vi "LCSS classification (edit).vi"(9 "cluster centers":string[](array[string])=["1 0 -1 1 -1 0 -4 1 -4 0 1", "2 0 -1 2 -1 0 -2 2 -2 0 2", "3 0 -3 3 -3 0 -2 3 -2 0 3", "4 0 -3 4 -3 0 -4 4 -4 0 4", "-1 1 -4 0 -4 4 -3 4 -4 0 -4 1 -1", "-1 2 -2 0 -2 3 -3 3 -2 0 -2 2 -1", "-4 1 -1 0 -1 2 -2 2 -1 0 -1 1 -4", "-4 4 -3 0 -3 3 -2 3 -3 0 -3 4 -4", "0 -4 1 -1 0 -3 3 -2 3 -3 0 -1 1 -4 0", "0 -4 4 -3 0 -1 2 -2 2 -1 0 -3 4 -4 0"], 11 "Patterns in":string[](array[string])=["0 4 0", "4 0 4", "0 4 0", "4 0 4", "0 4 0", "4 0 4", "0 4 0", "4 0 -2", "0 -2 3", "-2 3 0", "3 0 3", "0 3 0", "3 0 4", "0 4 0", "-2 0 1", "0 1 0", "1 0 -4", "0 -4 4", "-2 2 0", "2 0 -1", "0 -1 -4", "-1 -4 1", "-4 1 0", "1 0 3", "0 3 0", "-1 0 -1", "0 -1 2", "0 -1 1", "-1 1 0", "1 0 4", "0 4 0", "4 0 3", "0 3 -2", "3 -2 0", "-2 0 -2", "0 -2 3", "-2 3 -2", "3 -2 0", "-2 0 4", "0 4 0", "4 0 -2", "0 -2 2", "2 -1 0", "-1 0 4", "0 4 0", "4 0 2", "0 2 0", "2 0 -2", "0 -2 0", "1 -1 0", "-1 0 3", "0 3 0", "3 0 -4", "0 -4 4", "-4 4 -4", "4 -4 0", "2 -1 0", "-1 0 3", "0 3 -2", "3 -2 0", "-2 0 -3", "0 -3 0", "-3 0 3", "0 3 0", "3 0 -3", "0 -3 0", "0 4 0", "4 0 4", "0 4 -4", "4 -4 1", "-4 1 -1", "1 -1 0", "-1 0 -3", "0 -3 0", "-3 0 1", "0 1 -4", "1 -4 1", "-4 1 0", "1 0 4", "0 4 0", "4 0 -4", "0 -4 0", "-4 0 -4", "0 -4 4", "-4 4 -4", "4 -4 1", "0 -4 1", "-4 1 0", "1 0 -4", "0 -4 4", "0 4 0", "4 0 -2", "0 -2 2", "-2 2 -2", "2 -2 2", "-2 2 -2", "2 -2 2", "-2 2 -1", "2 -1 0", "-1 0 4", "0 4 0", "4 0 2", "0 2 0", "2 0 4", "0 4 0", "4 0 2", "0 2 -2", "2 -2 0", "-2 0 4", "1 0 -1", "0 -1 0", "-1 0 -1", "0 -1 0", "-1 0 1", "0 1 -1", "-2 2 -2", "2 -2 3", "1 0 -1", "0 -1 0", "-1 0 -1", "0 -1 2", "-1 2 0", "2 0 2", "0 2 -2", "2 -2 0", "-2 0 -4", "0 -4 0", "-2 2 0", "2 0 3", "0 3 -2", "3 -2 2", "1 -1 0", "-1 0 3", "0 4 0", "-2 0 1", "0 1 -4", "1 -4 0", "-4 0 -3", "0 -3 0", "1 0 -1", "0 -1 2", "-1 2 -1", "2 -1 1", "-1 1 -4", "-2 0 -1", "0 -1 1", "0 3 0", "3 0 3", "0 3 0", "3 0 3", "0 3 -2", "-4 0 -4", "0 -4 4", "0 4 0", "4 0 -4", "0 -4 0", "-4 0 -4", "-2 2 0", "2 0 4", "0 4 -4", "4 -4 0", "-4 0 2", "0 2 -2"]) -> (0 "Assigned cluster (0) unassigned":string[](array[string]), 1 "patterns in, distance values":string[][](array[string]), 2 "Assigned cluster 2nd method":string[](array[string]), 3 "Cluster element count":i32[](array[numeric]), 4 "Assigned cluster 3rd method 2":string[](array[string]))   [LabVIEW 2014]
panel:
  out "x = y?":bool[](array[boolean])
  out "Assigned cluster (0) unassigned 2":string[](array[string])
  out "Array 4":dbl[][](array[numeric])
  out "Array 3":dbl[][](array[numeric])
  out "Array 2":dbl[][](array[numeric])
  out "Array":dbl[][](array[numeric])
  out "L cluster centers":i32[](array[numeric])
  out "L sample":i32[](array[numeric])
  out "appended array":string[][](array[string])
  out "Distance values (LCS)":dbl[][](array[numeric])
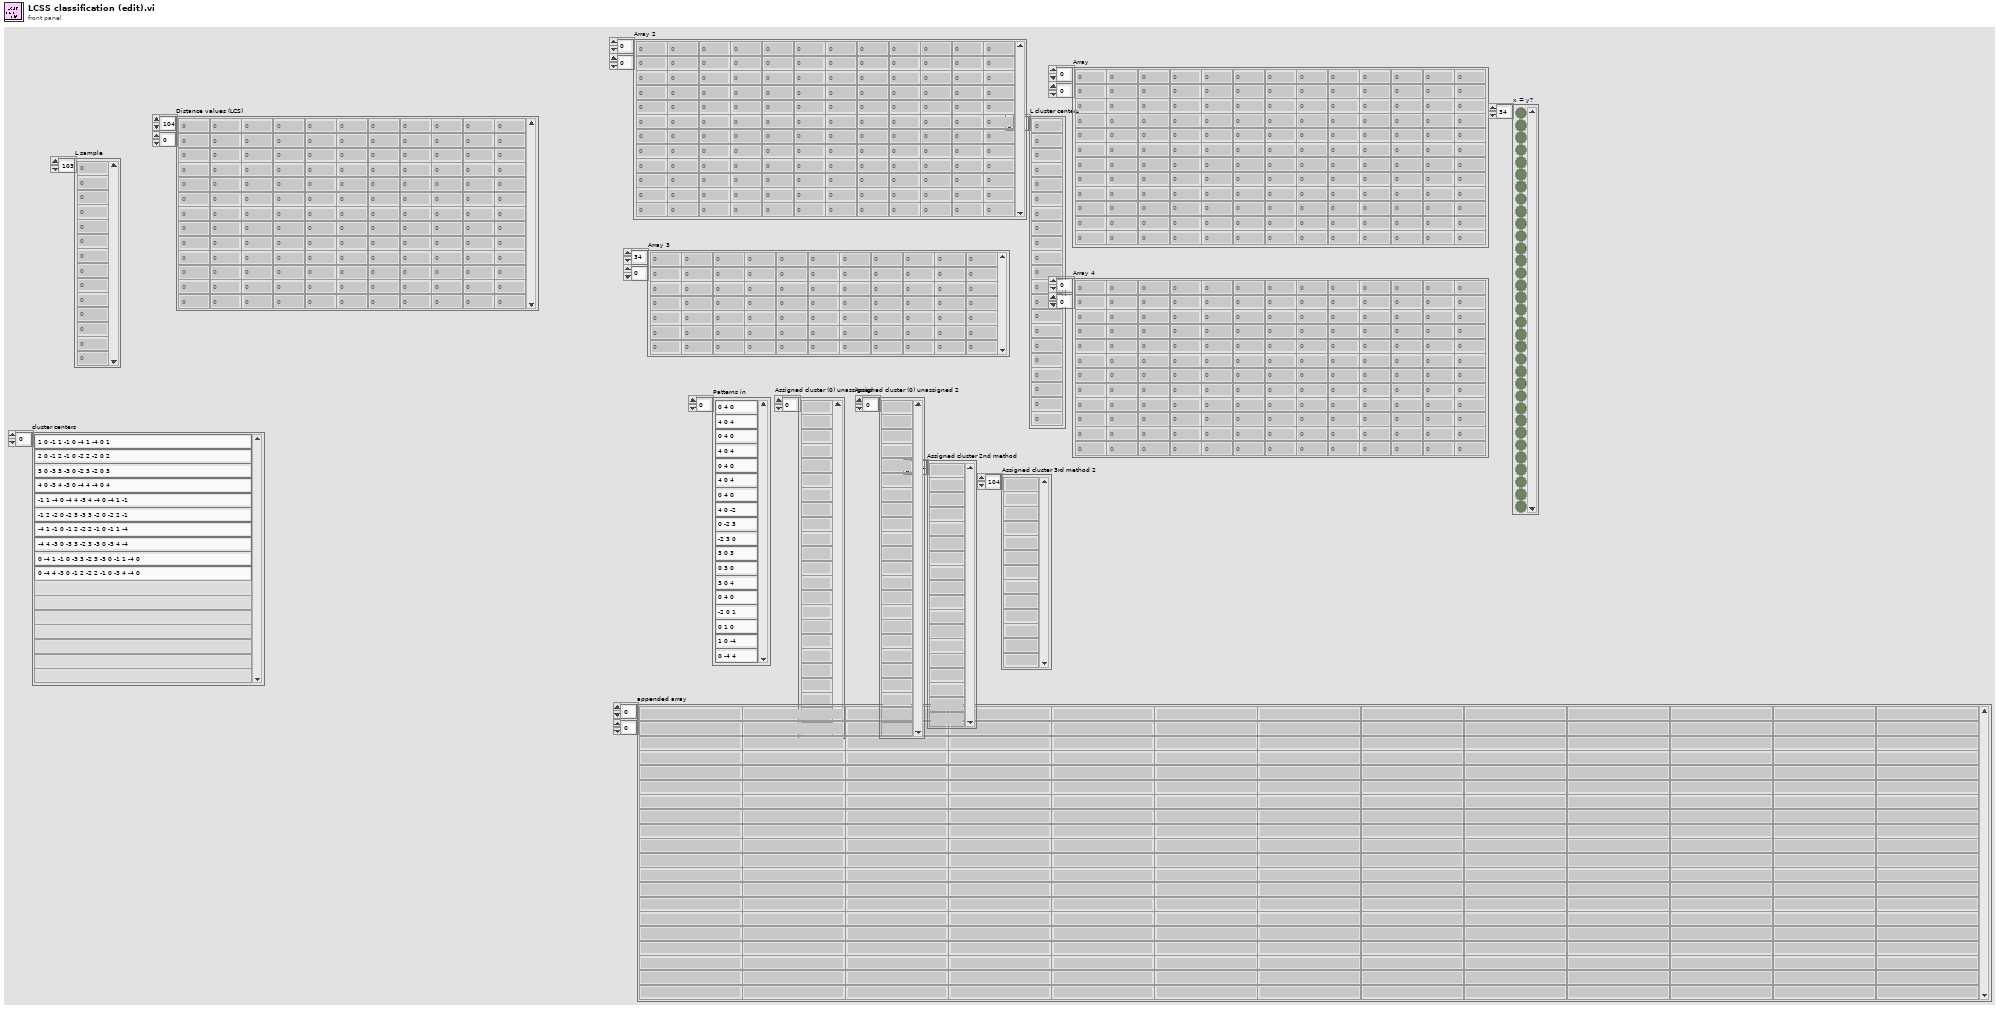
[diagram p1: front panel]
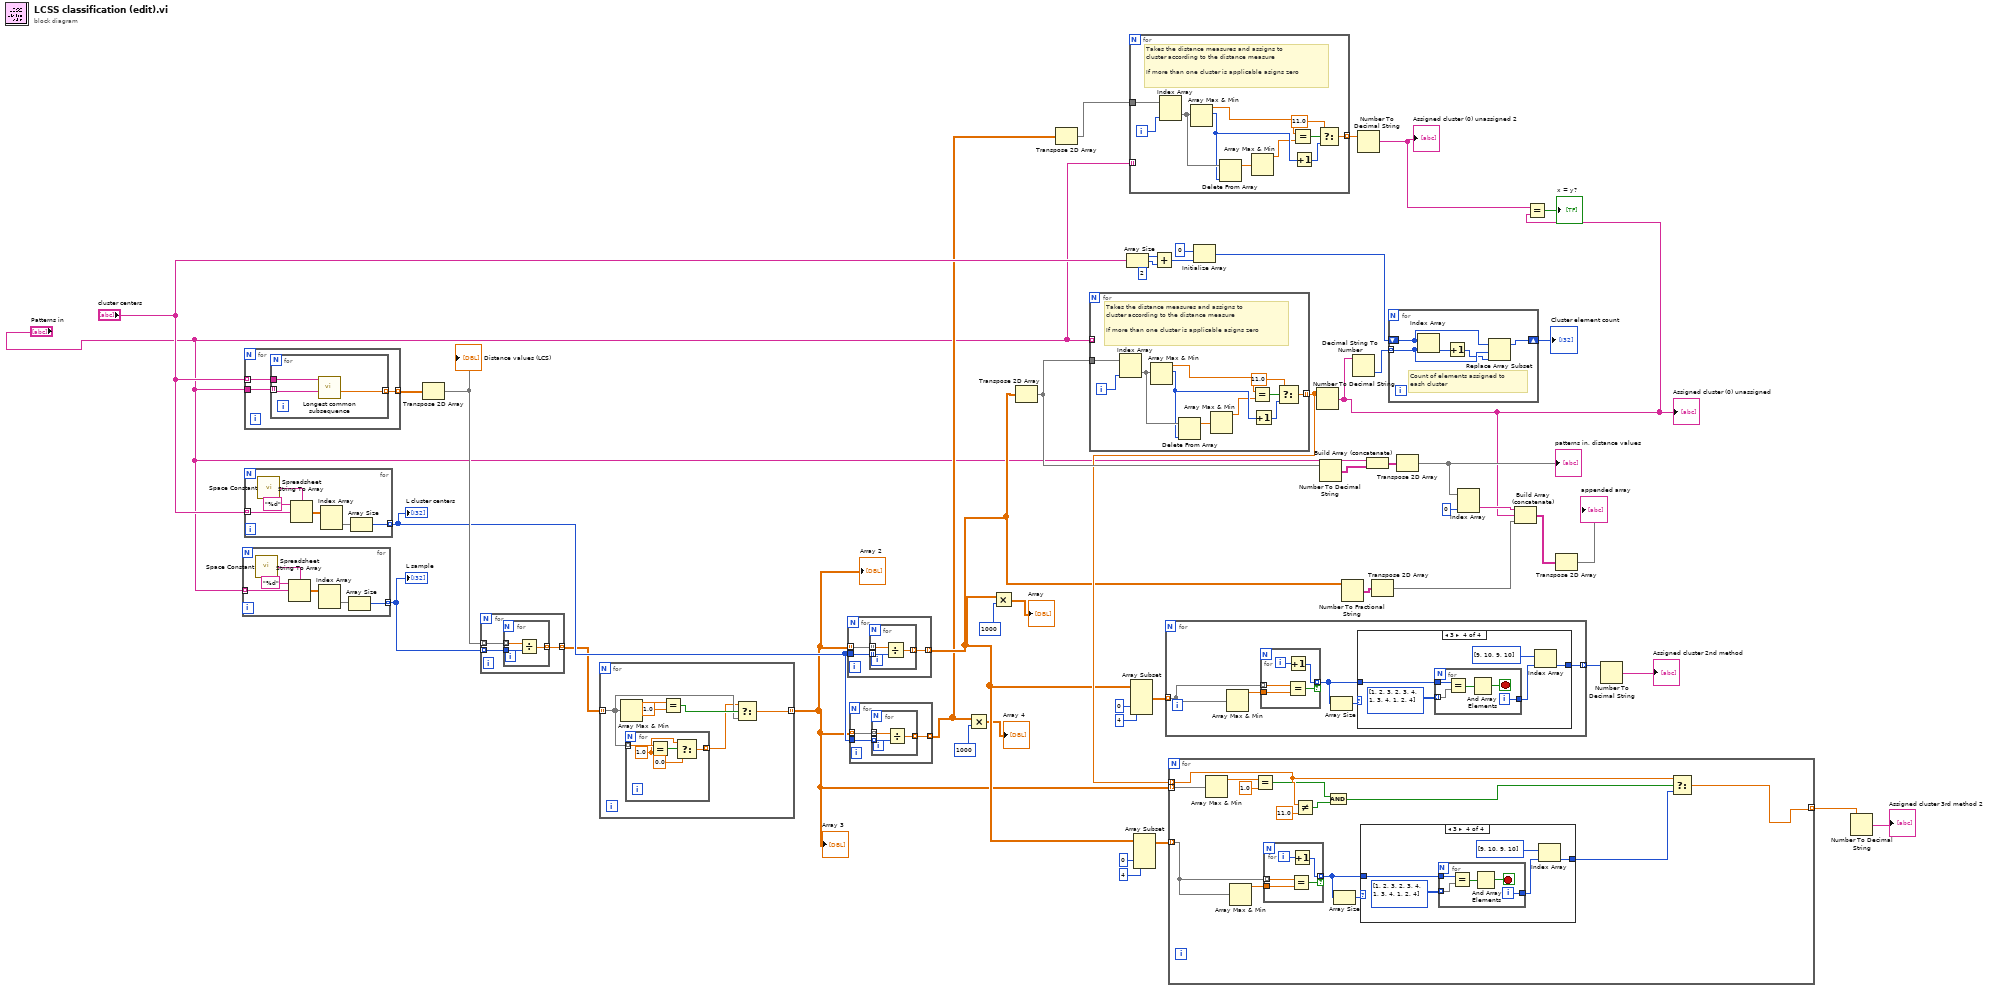
[diagram p0: block diagram]
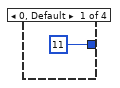
[diagram p2: hidden frame]
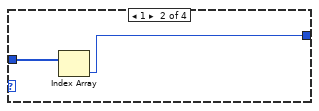
[diagram p3: hidden frame]
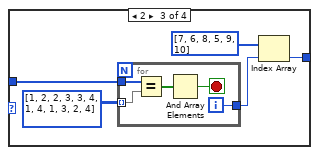
[diagram p4: hidden frame]
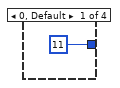
[diagram p5: hidden frame]
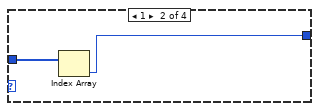
[diagram p6: hidden frame]
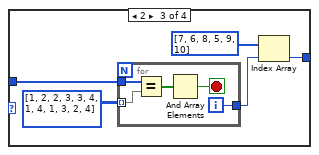
[diagram p7: hidden frame]
diagram:
  n1 = for {
    tunnel: "Patterns in" -> [w52] mode=indexing
    tunnel: [w48] -> w18 mode=indexing
    n2 = call <vilib>:"Space Constant.vi"() -> ("String"=w53:string)
    n3 = Spreadsheet String To Array(delimiter (Tab)=w53, format string="%d", spreadsheet string=w52) -> (array=w50:dbl[][])  [unwired: 1 in]
    n4 = Index Array(array=w50) -> (element=w49:dbl[])  [unwired: 2 in]
    n5 = Array Size(array=w49) -> (size(s)=w48:i32)
  }
  "L sample" <- w18
  n6 = for {
    tunnel: "cluster centers" -> [w56] mode=indexing
    tunnel: [w55] -> w30 mode=indexing
    tunnel: "Patterns in" -> [w54]
    n7 = for {
      tunnel: w54 -> [w58] mode=indexing
      tunnel: w56 -> [w59]
      tunnel: [w57] -> w55 mode=indexing
      n8 = call "Longest common subsequence.vi"("Pattern 2 COLUMN(0)"=w58, "Pattern 1 ROW(0)"=w59) -> ("LCS length"=w57:dbl)  [unwired: 8 in, 1 out]
    }
  }
  n9 = for {
    tunnel: "cluster centers" -> [w64] mode=indexing
    tunnel: [w60] -> w12 mode=indexing
    n10 = call <vilib>:"Space Constant.vi"() -> ("String"=w65:string)
    n11 = Spreadsheet String To Array(delimiter (Tab)=w65, format string="%d", spreadsheet string=w64) -> (array=w62:dbl[][])  [unwired: 1 in]
    n12 = Index Array(array=w62) -> (element=w61:dbl[])  [unwired: 2 in]
    n13 = Array Size(array=w61) -> (size(s)=w60:i32)
  }
  "L cluster centers" <- w12
  n14 = Transpose 2D Array(2D array=w30) -> (transposed array=w19:dbl[][])
  "Distance values (LCS)" <- w19
  n15 = for {
    tunnel: w19 -> [w68] mode=indexing
    tunnel: w18 -> [w67] mode=indexing
    tunnel: [w66] -> w2 mode=indexing
    n16 = for {
      tunnel: w68 -> [w71] mode=indexing
      tunnel: w67 -> [w70]
      tunnel: [w69] -> w66 mode=indexing
      n17 = Divide(x=w71, y=w70) -> (x/y=w69:dbl)
    }
  }
  n18 = for {
    tunnel: w2 -> [w73] mode=indexing
    tunnel: [w74] -> w1 mode=indexing
    n19 = Array Max & Min(array=w73) -> (max value=w77:dbl)  [unwired: 3 out]
    n20 = for {
      tunnel: w73 -> [w82] mode=indexing
      tunnel: [w78] -> w72 mode=indexing
      w80 = 1.0 ("y")
      n21 = Equal?(x=w82, y=w80) -> (x = y?=w81:bool)
      n22 = Select(t=w80, s=w81, f=0.0) -> (s? t:f=w78:dbl)
    }
    n23 = Equal?(x=w77, y=1.0) -> (x = y?=w75:bool)
    n24 = Select(t=w72, s=w75, f=w73) -> (s? t:f=w74:dbl[])
  }
  "Array 2" <- w1
  "Array 3" <- w1
  n25 = for {
    tunnel: w1 -> [w85] mode=indexing
    tunnel: w12 -> [w84]
    tunnel: [w83] -> w16 mode=indexing
    n26 = for {
      tunnel: w85 -> [w88] mode=indexing
      tunnel: w84 -> [w86] mode=indexing
      tunnel: [w87] -> w83 mode=indexing
      n27 = Divide(x=w88, y=w86) -> (x/y=w87:dbl)
    }
  }
  n28 = for {
    tunnel: w1 -> [w91] mode=indexing
    tunnel: w12 -> [w90]
    tunnel: [w89] -> w7 mode=indexing
    n29 = for {
      tunnel: w91 -> [w94] mode=indexing
      tunnel: w90 -> [w92] mode=indexing
      tunnel: [w93] -> w89 mode=indexing
      n30 = Divide(x=w94, y=w92) -> (x/y=w93:dbl)
    }
  }
  n31 = Multiply(x=w7, y=1000) -> (x*y=→"Array 4":dbl[][])
  n32 = Multiply(x=w16, y=1000) -> (x*y=→"Array":dbl[][])
  n33 = Transpose 2D Array(2D array=w16) -> (transposed array=w32:dbl[][])
  n34 = Transpose 2D Array(2D array=w7) -> (transposed array=w8:dbl[][])
  n35 = for {
    tunnel: "Patterns in" -> [_] mode=indexing
    tunnel: w32 -> [w105]
    tunnel: [w95] -> w17 mode=indexing
    i -> [w104]
    # "Takes the distance measures and assigns to \ncluster according to the distance measure\n\nIf more than one cluster is applicable asigns zero"
    n36 = Index Array(array=w105, index (col)=w104) -> (element=w99:dbl[])  [unwired: 1 in]
    n37 = Array Max & Min(array=w99) -> (max value=w98:dbl, max index (indices)=w97:i32)  [unwired: 2 out]
    n38 = Delete From Array(array=w99, index=w97) -> (array with subset deleted=w103:dbl[])  [unwired: 1 in, 1 out]
    n39 = Array Max & Min(array=w103) -> (max value=w96:dbl)  [unwired: 3 out]
    n40 = Equal?(x=w98, y=w96) -> (x = y?=w102:bool)
    n41 = Increment(x=w97) -> (x+1=w100:i32)
    n42 = Select(t=11.0, s=w102, f=w100) -> (s? t:f=w95:dbl)
  }
  n43 = Array Size(array="cluster centers") -> (size(s)=w42:i32)
  n44 = for {
    tunnel: w8 -> [w116]
    tunnel: [w106] -> w9 mode=indexing
    tunnel: "Patterns in" -> [_] mode=indexing
    i -> [w115]
    # "Takes the distance measures and assigns to \ncluster according to the distance measure\n\nIf more than one cluster is applicable asigns zero"
    n45 = Index Array(array=w116, index (col)=w115) -> (element=w110:dbl[])  [unwired: 1 in]
    n46 = Array Max & Min(array=w110) -> (max value=w109:dbl, max index (indices)=w108:i32)  [unwired: 2 out]
    n47 = Delete From Array(array=w110, index=w108) -> (array with subset deleted=w114:dbl[])  [unwired: 1 in, 1 out]
    n48 = Array Max & Min(array=w114) -> (max value=w107:dbl)  [unwired: 3 out]
    n49 = Equal?(x=w109, y=w107) -> (x = y?=w113:bool)
    n50 = Increment(x=w108) -> (x+1=w111:i32)
    n51 = Select(t=11.0, s=w113, f=w111) -> (s? t:f=w106:dbl)
  }
  n52 = Array Subset(array=w16, index (col)=0 ("index"), length (col)=4 ("length")) -> (w27:dbl[][])  [unwired: 2 in]
  n53 = Array Subset(array=w16, index (col)=0 ("index"), length (col)=4 ("length")) -> (w23:dbl[][])  [unwired: 2 in]
  n54 = Add(x=2, y=w42) -> (x+y=w41:i32)
  n55 = for {
    tunnel: w27 -> [w121] mode=indexing
    tunnel: [w117] -> w26 mode=indexing
    n56 = Array Max & Min(array=w121) -> (max value=w120:dbl)  [unwired: 3 out]
    n57 = for {
      tunnel: w121 -> [w149] mode=indexing
      tunnel: w120 -> [w148]
      tunnel: [w145] -> w118 mode=indexing if=w147
      i -> [w146]
      n58 = Equal?(x=w149, y=w148) -> (x = y?=w147:bool)
      n59 = Increment(x=w146) -> (x+1=w145:i32)
    }
    n60 = Array Size(array=w118) -> (size(s)=w119:i32)
    n61 = case shown="3" w119 {
      tunnel: w118 -> [_ w124 w128 w139]
      tunnel: [11 w123 w126 w138] -> w117
      frame 0, Default {
      }
      frame 1 {
        n62 = Index Array(array=w124) -> (element=w123:i32)  [unwired: 1 in]
      }
      frame 2 {
        n63 = for {
          tunnel: i32[][] [[1, 2], [2, 3], [3, 4], [1, 4], [1, 3], [2, 4]] -> [w134] mode=indexing
          tunnel: w128 -> [w133]
          tunnel: [w131] -> w125
          i -> [w131]
          stop <- w130 stop-if-true
          n64 = Equal?(x=w133, y=w134) -> (x = y?=w132:bool[])
          n65 = And Array Elements(Boolean array=w132) -> (logical AND=w130:bool)
        }
        n66 = Index Array(array=i32[] [7, 6, 8, 5, 9, 10], index=w125) -> (element=w126:i32)
      }
      frame 3 {
        n67 = for {
          tunnel: i32[][] [[1, 2, 3], [2, 3, 4], [1, 3, 4], [1, 2, 4]] -> [w144] mode=indexing
          tunnel: w139 -> [w143]
          tunnel: [w141] -> w137
          i -> [w141]
          stop <- w140 stop-if-true
          n68 = Equal?(x=w143, y=w144) -> (x = y?=w142:bool[])
          n69 = And Array Elements(Boolean array=w142) -> (logical AND=w140:bool)
        }
        n70 = Index Array(array=i32[] [9, 10, 9, 10], index=w137) -> (element=w138:i32)
      }
    }
  }
  n71 = for {
    tunnel: w23 -> [w163] mode=indexing
    tunnel: [w155] -> w24 mode=indexing
    tunnel: w17 -> [w153] mode=indexing
    tunnel: w1 -> [w159] mode=indexing
    n72 = Array Max & Min(array=w159) -> (max value=w158:dbl)  [unwired: 3 out]
    n73 = Array Max & Min(array=w163) -> (max value=w162:dbl)  [unwired: 3 out]
    n74 = Equal?(x=w158, y=1.0 ("t")) -> (x = y?=w151:bool)
    n75 = for {
      tunnel: w163 -> [w191] mode=indexing
      tunnel: w162 -> [w190]
      tunnel: [w187] -> w160 mode=indexing if=w189
      i -> [w188]
      n76 = Equal?(x=w191, y=w190) -> (x = y?=w189:bool)
      n77 = Increment(x=w188) -> (x+1=w187:i32)
    }
    n78 = Not Equal?(x=w153, y=11.0 ("t")) -> (x != y?=w152:bool)
    n79 = And(x=w151, y=w152) -> (x .and. y?=w150:bool)
    n80 = Array Size(array=w160) -> (size(s)=w161:i32)
    n81 = case shown="3" w161 {
      tunnel: w160 -> [_ w166 w170 w181]
      tunnel: [11 w165 w168 w180] -> w156
      frame 0, Default {
      }
      frame 1 {
        n82 = Index Array(array=w166) -> (element=w165:i32)  [unwired: 1 in]
      }
      frame 2 {
        n83 = for {
          tunnel: i32[][] [[1, 2], [2, 3], [3, 4], [1, 4], [1, 3], [2, 4]] -> [w176] mode=indexing
          tunnel: w170 -> [w175]
          tunnel: [w173] -> w167
          i -> [w173]
          stop <- w172 stop-if-true
          n84 = Equal?(x=w175, y=w176) -> (x = y?=w174:bool[])
          n85 = And Array Elements(Boolean array=w174) -> (logical AND=w172:bool)
        }
        n86 = Index Array(array=i32[] [7, 6, 8, 5, 9, 10], index=w167) -> (element=w168:i32)
      }
      frame 3 {
        n87 = for {
          tunnel: i32[][] [[1, 2, 3], [2, 3, 4], [1, 3, 4], [1, 2, 4]] -> [w186] mode=indexing
          tunnel: w181 -> [w185]
          tunnel: [w183] -> w179
          i -> [w183]
          stop <- w182 stop-if-true
          n88 = Equal?(x=w185, y=w186) -> (x = y?=w184:bool[])
          n89 = And Array Elements(Boolean array=w184) -> (logical AND=w182:bool)
        }
        n90 = Index Array(array=i32[] [9, 10, 9, 10], index=w179) -> (element=w180:i32)
      }
    }
    n91 = Select(t=w153, s=w150, f=w156) -> (s? t:f=w155:dbl)
  }
  n92 = Initialize Array(0 ("index"), w41) -> (w40:i32[])
  n93 = Number To Decimal String(number=w17) -> (decimal integer string=w4:string[])  [unwired: 1 in]
  "Assigned cluster (0) unassigned" <- w4
  n94 = Number To Decimal String(number=w32) -> (decimal integer string=w44:string[][])  [unwired: 1 in]
  n95 = Number To Fractional String(number=w16) -> (F-format string=w33:string[][])  [unwired: 3 in]
  n96 = Decimal String To Number(string=w4) -> (number=w46:i32[])  [unwired: 2 in, 1 out]
  n97 = Number To Decimal String(number=w9) -> (decimal integer string=w5:string[])  [unwired: 1 in]
  "Assigned cluster (0) unassigned 2" <- w5
  n98 = Build Array (concatenate)("Patterns in", w44) -> (w47:string[][])
  n99 = Transpose 2D Array(2D array=w33) -> (transposed array=w34:string[][])
  n100 = for {
    tunnel: w46 -> [w194] mode=indexing
    shift-right: [w192] -> w45
    shift-left: w40 -> [w195]
    # "Count of elements assigned to \neash cluster"
    n101 = Index Array(array=w195, index=w194) -> (element=w196:i32)
    n102 = Increment(x=w196) -> (x+1=w193:i32)
    n103 = Replace Array Subset(array=w195, new element=w193, index=w194) -> (w192:i32[])
  }
  "Cluster element count" <- w45
  n104 = Transpose 2D Array(2D array=w47) -> (transposed array=w39:string[][])
  "patterns in, distance values" <- w39
  n105 = Index Array(array=w39, index (col)=0 ("disabled index (col)")) -> (element=w37:string[])  [unwired: 1 in]
  n106 = Build Array (concatenate)(w37, w4, w34) -> (w36:string[][])
  n107 = Equal?(x=w5, y=w4) -> (x = y?=→"x = y?":bool[])
  n108 = Transpose 2D Array(2D array=w36) -> (transposed array=→"appended array":string[][])
  n109 = Number To Decimal String(number=w26) -> (decimal integer string=→"Assigned cluster 2nd method":string[])  [unwired: 1 in]
  n110 = Number To Decimal String(number=w24) -> (decimal integer string=→"Assigned cluster 3rd method 2":string[])  [unwired: 1 in]
